vi "IS Open-Create Bucket.vi"(6 "Tags (Optional: Auto-Populates \"labview\")":string[](array[string]), 7 "Operation (0: open)":enum16{"open", "create"}(ring), 8 "error in (no error)":errorcluster, 9 "Bucket Name (Optional)":string="LabVIEW-Created Bucket", 10 "Bucket Key (Optional)":string, 11 "IS Session In":T2={"Access Key"="", "HTTP Client Handle"=refnum}) -> (0 "error IO":errorcluster, 2 "IS Bucket Session":T1, 3 "IS Session Out":T2)   [LabVIEW 2018]
doc: "This VI either opens or creates an Initial State Bucket. When opening an existing bucket, you must provide a valid Bucket Key. When creating a new bucket, you can provide a key or let a random key get generated. In addition, you can tag your bucket with user-defined tags. The VI automatically tags new buckets with \"labview.\" This VI does the proper HTTP POST to create a new Bucket in your Initial State accout. In both open and create cases, the resulting Bucket Key is added to the header information of the Initial State HTTP Request."
uses:
  Controls/IS Session.ctl
  <vilib>/httpClient/ClientHandle.ctl
  Controls/IS Bucket Session.ctl
  <vilib>/httpClient/POSTBuffer.vi
  <vilib>/httpClient/LabVIEWHTTPClient.lvlib
panel:
  out "appended array":string[](array[string])
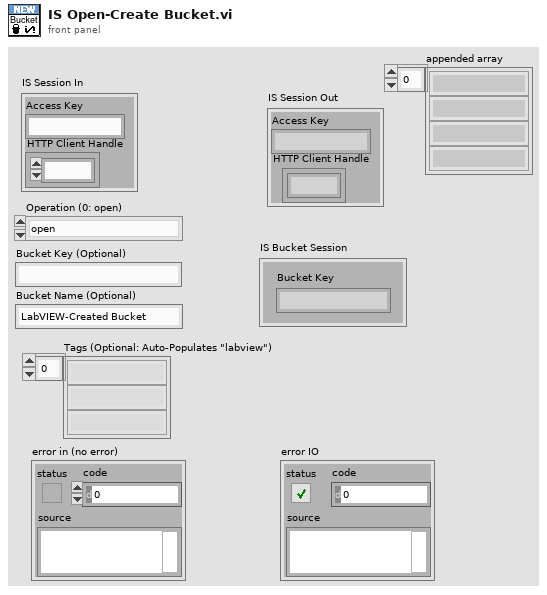
[diagram p1: front panel]
types:
  T1 = typedef "IS Bucket Session.ctl" = cluster{"Bucket Key":string}
  T2 = typedef "IS Session.ctl" = cluster{"Access Key":string, "HTTP Client Handle":T3}
  T3 = typedef "LabVIEWHTTPClient.lvlib/ClientHandle.ctl" = refnum<k1>
  T4 = cluster{"bucketName":string, "bucketKey":string, "tags":string[]}
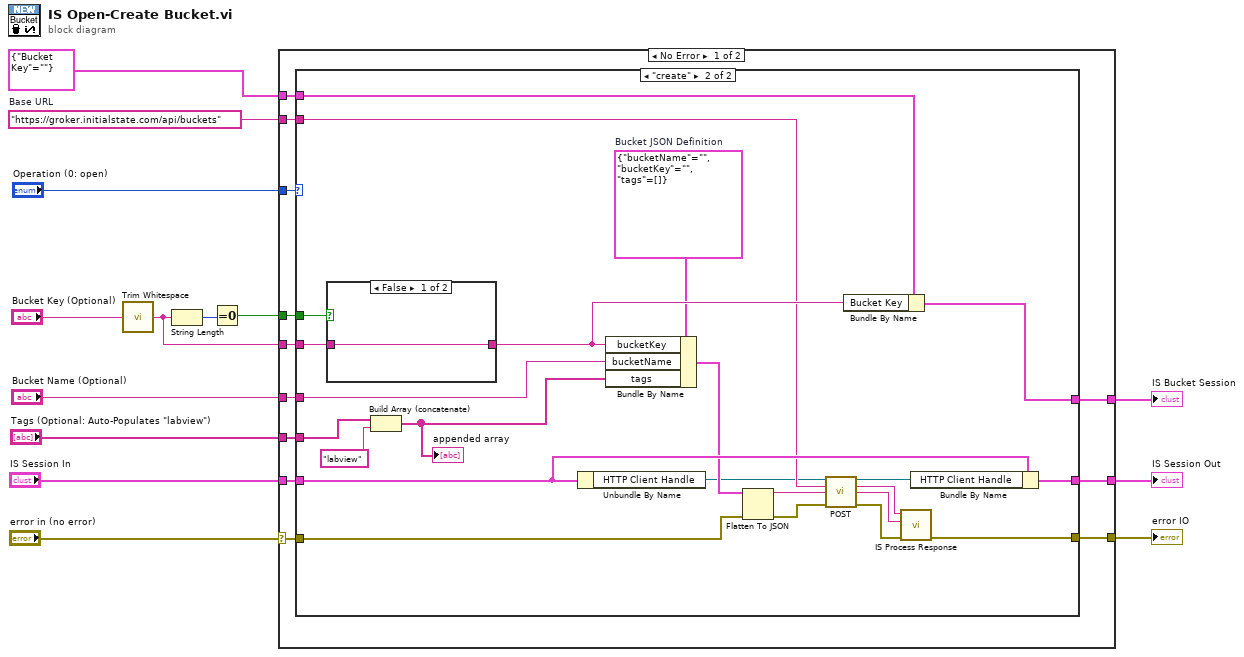
[diagram p0: block diagram]
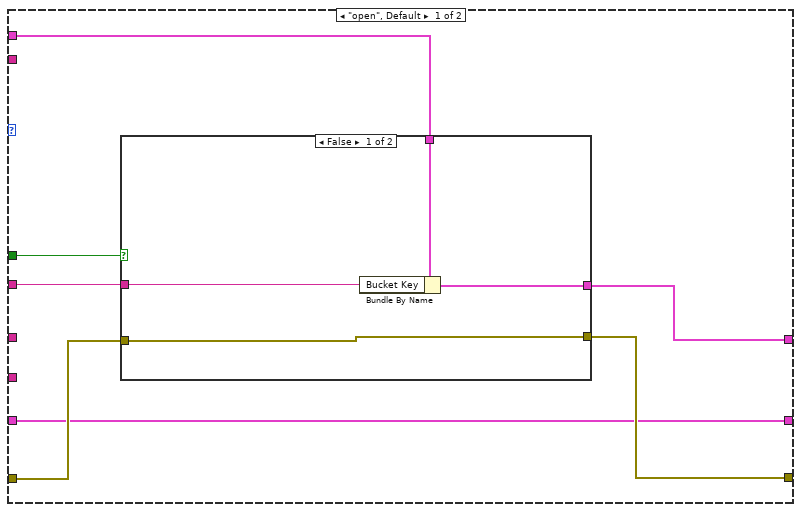
[diagram p2: hidden frame]
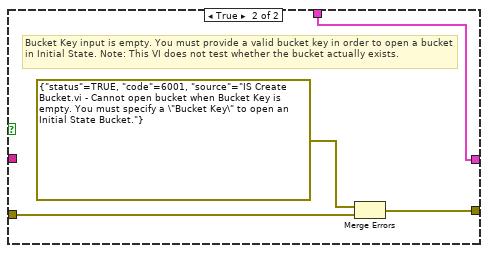
[diagram p3: hidden frame]
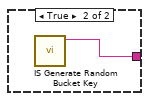
[diagram p4: hidden frame]
diagram:
  w6 = "https://groker.initialstate.com/api/buckets"  # Base URL
  n1 = call <vilib>:"Trim Whitespace.vi"("string"="Bucket Key (Optional)") -> ("trimmed string"=w8:string)  [unwired: 1 in]
  n2 = String Length(string=w8) -> (length=w11:i32)
  n3 = Equal To 0?(x=w11) -> (x = 0?=w10:bool)
  n4 = case shown="No Error" "error in (no error)" {
    selector: "error in (no error)" -> [w16 w69]
    tunnel: "IS Session In" -> [w26 w68]
    tunnel: [w25 w68] -> w13
    tunnel: [w24 w69] -> w12
    tunnel: w10 -> [w23 _]
    tunnel: w8 -> [w22 _]
    tunnel: [w21 w67] -> w7
    tunnel: w6 -> [w20 _]
    tunnel: "Bucket Name (Optional)" -> [w19 _]
    tunnel: "Operation (0: open)" -> [w18 _]
    tunnel: T1 {"Bucket Key"=""} ("IS Bucket Session") -> [w17 w67]
    tunnel: "Tags (Optional: Auto-Populates \"labview\")" -> [w15 _]
    frame No Error {
      n5 = case shown="\"create\"" w18 {
        tunnel: w26 -> [w27 w64]
        tunnel: w16 -> [w28 w50]
        tunnel: [w27 w63] -> w25
        tunnel: [w29 w48] -> w24
        tunnel: w23 -> [w30 w62]
        tunnel: w22 -> [w32 w61]
        tunnel: [w31 w59] -> w21
        tunnel: w20 -> [_ w58]
        tunnel: w19 -> [_ w57]
        tunnel: w17 -> [w33 w56]
        tunnel: w15 -> [_ w44]
        frame "open", Default {
          n6 = case shown="False" w30 {
            tunnel: w33 -> [w37 w38]
            tunnel: w32 -> [w36 _]
            tunnel: [w35 w38] -> w31
            tunnel: w28 -> [w34 w40]
            tunnel: [w34 w39] -> w29
            frame False {
              n7 = Bundle By Name(cluster=w37, "Bucket Key"=w36) -> (w35:T1)
            }
            frame True {
              # "Bucket Key input is empty. You must provide a valid bucket key in order to open a bucket in Initial State. Note: This VI does not test whether the bucket actually exists."
              n8 = Merge Errors(errorcluster {"status"=TRUE, "code"=6001, "source"="IS Create Bucket.vi - Cannot open bucket when Bucket Key is empty. You must specify a \"Bucket Key\" to open an Initial State Bucket."} ("error in (no error)"), w40) -> (w39:errorcluster)
            }
          }
        }
        frame "create" {
          w45 = T4 {"bucketName"="", "bucketKey"="", "tags"=[]}  # Bucket JSON Definition
          n9 = case shown="False" w62 {
            tunnel: [w65 w66] -> w60
            tunnel: w61 -> [w65 _]
            frame False {
            }
            frame True {
              n10 = call "IS Generate Random Bucket Key.vi"() -> ("Random Bucket Key String"=w66:string)  [unwired: 11 in]
            }
          }
          n11 = Build Array (concatenate)(w44, "labview" ("tag")) -> (w42:string[])
          "appended array" <- w42
          n12 = Unbundle By Name(w64) -> ("HTTP Client Handle"=w51:T3)
          n13 = Bundle By Name(cluster=w45, "bucketKey"=w60, "bucketName"=w57, "tags"=w42) -> (w54:T4)
          n14 = Flatten To JSON(anything=w54, error in (no error)=w50) -> (JSON string=w52:string, 11:w53:errorcluster)  [unwired: 1 in]
          n15 = call-poly <vilib>:"POST.vi"("client handle"=w51, "url"=w58, "buffer"=w52, "error in (no error)"=w53) -> ("client handle out"=w55:T3, "headers"=w47:string, "body"=w46:string, "error out"=w49:errorcluster)  [unwired: 8 in]
          n16 = Bundle By Name(cluster=w56, "Bucket Key"=w60) -> (w59:T1)
          n17 = call "IS Process Response.vi"("Error In (no error)"=w49, "Response Body"=w46, "Response Headers"=w47) -> ("Error Out"=w48:errorcluster)  [unwired: 7 in, 1 out]
          n18 = Bundle By Name(cluster=w64, "HTTP Client Handle"=w55) -> (w63:T2)
        }
      }
    }
    frame Error {
    }
  }
  "IS Session Out" <- w13
  "error IO" <- w12
  "IS Bucket Session" <- w7
